vi "createYi.vi"(9 "Min":dbl, 10 "Max":dbl, 11 "delta":dbl) -> (2 "max value":dbl, 3 "Array":dbl[](array[numeric]))   [LabVIEW 2013]
uses:
  NI_AALBase.lvlib
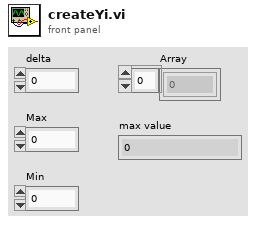
[diagram p1: front panel]
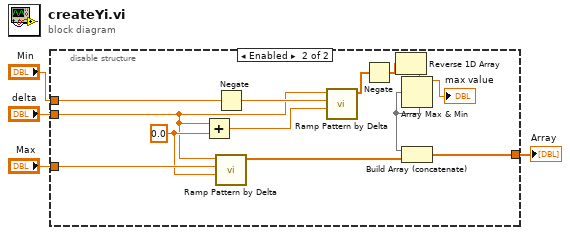
[diagram p0: block diagram]
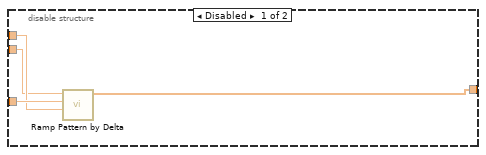
[diagram p2: hidden frame]
diagram:
  n1 = disable-structure shown="Enabled" {
    disable-tunnel: "Max" -> [w8 w20]
    disable-tunnel: [w7 w19] -> w2
    disable-tunnel: "Min" -> [w6 w16]
    disable-tunnel: "delta" -> [w5 w13]
    frame Disabled {
      n2 = call "Ramp Pattern by Delta.vi"("start"=w6, "end"=w8, "delta"=w5) -> ("Ramp Pattern"=w7:dbl[])  [unwired: 6 in, 2 out]
    }
    frame Enabled {
      w14 = 0.0 ("start")
      n3 = Add(x=w13, y=w14) -> (x+y=w12:dbl)
      n4 = Negate(x=w16) -> (-x=w15:dbl)
      n5 = call "Ramp Pattern by Delta.vi"("start"=w14, "end"=w20, "delta"=w13) -> ("Ramp Pattern"=w18:dbl[])  [unwired: 6 in, 2 out]
      n6 = call "Ramp Pattern by Delta.vi"("start"=w12, "end"=w15, "delta"=w13) -> ("Ramp Pattern"=w11:dbl[])  [unwired: 6 in, 2 out]
      n7 = Negate(x=w11) -> (-x=w10:dbl[])
      n8 = Reverse 1D Array(array=w10) -> (reversed array=w9:dbl[])
      n9 = Array Max & Min(array=w9) -> (max value=→"max value":dbl)  [unwired: 3 out]
      n10 = Build Array (concatenate)(w9, w18) -> (w19:dbl[])
    }
  }
  "Array" <- w2
